vi "usrp clock get sensor names.vi"(8 "error in (no error)":errorcluster, 9 "sensor_names_out":u64, 10 "board":u64, 11 "h":u64) -> (0 "error out":errorcluster, 1 "sensor_names_out out":u64, 3 "function return":u32(ring))   [LabVIEW 2023, in "uhd.lvlib"]
doc: "UHD_API uhd_error uhd_usrp_clock_get_sensor_names(\n uhd_usrp_clock_handle h, size_t board, uhd_string_vector_handle* sensor_names_out);"
uses:
  <userlib>/uhd/uhd.lvlib
  <userlib>/uhd/uhd.dll
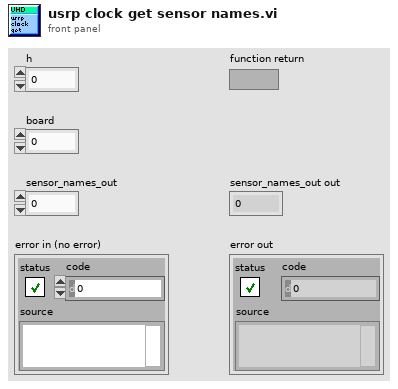
[diagram p1: front panel]
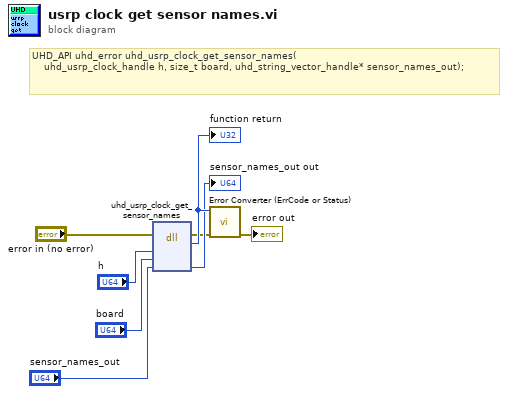
[diagram p0: block diagram]
diagram:
  # "UHD_API uhd_error uhd_usrp_clock_get_sensor_names(\n    uhd_usrp_clock_handle h, size_t board, uhd_string_vector_handle* sensor_names_out);"
  n1 = dll-call lib="C:/Program Files/National Instruments/LabVIEW 2023/user.lib/uhd/uhd.*" fn="uhd_usrp_clock_get_sensor_names"(error in="error in (no error)", "h"="h", "board"="board", "sensor_names_out"="sensor_names_out") -> (error out=w2:errorcluster, w8:u32, "sensor_names_out"=→"sensor_names_out out":u64)  [unwired: 4 in, 1 out]
  "function return" <- w8
  n2 = call <userlib>:"Error Converter (ErrCode or Status).vi"("error in (no error)"=w2, "error code"=w8) -> ("error out"=→"error out":errorcluster)  [unwired: 9 in]
